vi "numero_rand_1_10 _modi.vi"() -> ()   [LabVIEW 2020]
panel:
  out "valor del temporizador en mili 2":u32
  in  "millisecond timer value":u32
  in  "stop":bool
  out "number (0 to 1)":dbl
  out "I":i32
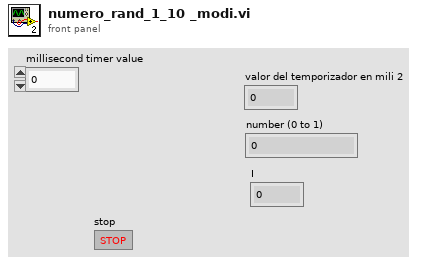
[diagram p1: front panel]
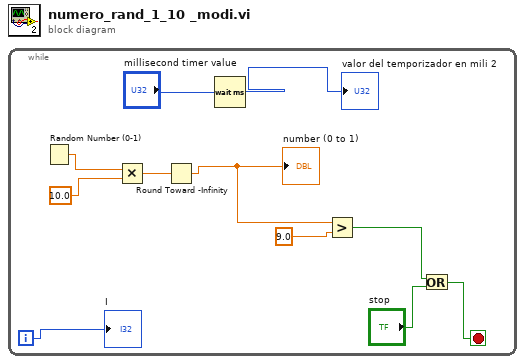
[diagram p0: block diagram]
diagram:
  n1 = while {
    i -> [w10]
    stop <- w3 stop-if-true
    n2 = Random Number (0-1)() -> (number: 0 to 1=w8:dbl)
    n3 = Multiply(x=w8, y=10.0 ("number (0 to 1)")) -> (x*y=w7:dbl)
    n4 = Round Toward -Infinity(1:w7) -> (0:w6:dbl)
    "number (0 to 1)" <- w6
    n5 = Wait (ms)(milliseconds to wait="millisecond timer value") -> (millisecond timer value=→"valor del temporizador en mili 2":u32)
    n6 = Greater?(x=w6, y=9.0 ("x")) -> (0:w4:bool)
    n7 = Or(x=w4, y="stop") -> (x .or. y?=w3:bool)
    "I" <- w10
  }
